vi "replace subvi from template.vi"() -> ()   [LabVIEW 2020]
uses:
  <vilib>/Utility/traverseref.llb/TRef TravTarget.ctl
  <vilib>/Utility/config.llb/Read Key (String).vi
  <vilib>/Utility/config.llb/NI_LVConfig.lvlib
  <vilib>/Utility/traverseref.llb/VI Scripting - Traverse.lvlib
panel:
  out "section exists?":bool
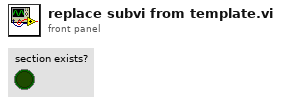
[diagram p1: front panel]
types:
  T1 = typedef "NI_LVConfig.lvlib/Config Data RefNum.ctl" = refnum<k1>
  T2 = typedef "TRef TravTarget.ctl" = enum16{"FP", "BD", "Other"}
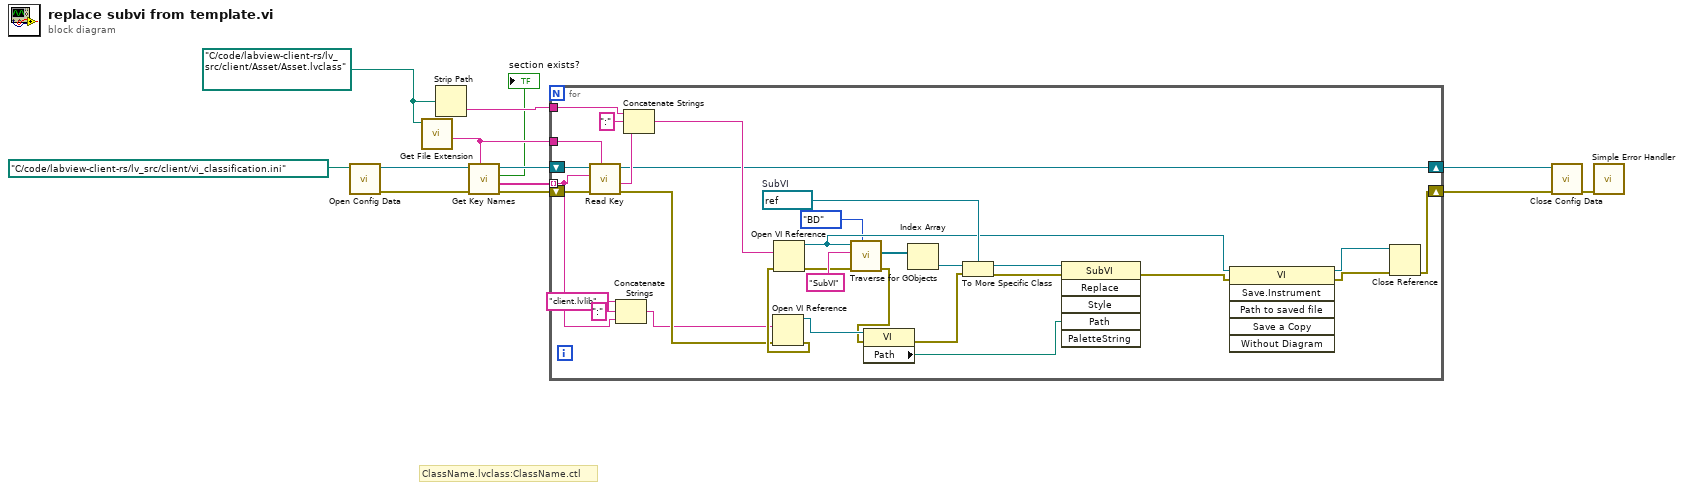
[diagram p0: block diagram]
diagram:
  w8 = path "C:/code/labview-client-rs/lv_src/client/Asset/Asset.lvclass" ("Path")
  # "ClassName.lvclass:ClassName.ctl"
  n1 = call <vilib>:"Open Config Data.vi"("configuration file path"=path "C:/code/labview-client-rs/lv_src/client/vi_classification.ini") -> ("error out"=w11:errorcluster, "refnum"=w1:T1)  [unwired: 8 in, 1 out]
  n2 = call <vilib>:"Get File Extension.vi"("file"=w8) -> ("filename without extension"=w7:string)  [unwired: 6 in, 4 out]
  n3 = Strip Path(path=w8) -> (name=w5:string)  [unwired: 1 out]
  n4 = call <vilib>:"Get Key Names.vi"("section"=w7, "error in (no error)"=w11, "refnum"=w1) -> ("error out"=w6:errorcluster, "key names"=w10:string[], "section exists?"=→"section exists?":bool, "refnum out"=w9:T1)  [unwired: 5 in]
  n5 = for {
    tunnel: w10 -> [w17] mode=indexing
    tunnel: w7 -> [w43]
    tunnel: w5 -> [w41]
    shift-right: [w25] -> w4
    shift-left: w9 -> [w44]
    shift-right: [w24] -> w3
    shift-left: w6 -> [w42]
    w34 = refnum<vi> refnum  # SubVI
    n6 = call-poly <vilib>:"Read Key.vi"("section"=w43, "error in (no error)"=w42, "key"=w17, "refnum"=w44) -> ("error out"=w18:errorcluster, "value"=w39:string, "refnum out"=w25:T1)  [unwired: 4 in, 1 out]
    n7 = Concatenate Strings("client.lvlib" ("string"), ":" ("string"), w17) -> (w14:string)
    n8 = Concatenate Strings(w41, ":" ("string"), w39) -> (w38:string)
    n9 = Open VI Reference(vi path=w14, error in (no error)=w18) -> (vi reference=w32:refnum<vi>, error out=w19:errorcluster)  [unwired: 4 in]
    n10 = Open VI Reference(vi path=w38, error in (no error)=w19) -> (vi reference=w29:refnum<vi>, error out=w20:errorcluster)  [unwired: 4 in]
    n11 = call <vilib>:"Traverse for GObjects.vi"("Traverse Target"=TRef_TravTarget."BD", "error in (no error)"=w20, "Class Name"="SubVI", "VI Refnum"=w29) -> ("error out"=w21:errorcluster, "References"=w36:refnum<vi>[])  [unwired: 4 in, 2 out]
    n12 = property class="VI"(reference=w32, error in=w21) -> (error out=w22:errorcluster, "Path"=w31:path)  [unwired: 1 out]
    n13 = Index Array(array=w36) -> (element=w35:refnum<vi>)  [unwired: 1 in]
    n14 = To More Specific Class(target class=w34, reference=w35, error in=w22) -> (specific class reference=w33:refnum<vi>, error out=w23:errorcluster)
    n15 = invoke class="SubVI" method="Replace"(reference=w33, error in=w23, "Path"=w31) -> (error out=w30:errorcluster)  [unwired: 3 in, 5 out]
    n16 = invoke class="VI" method="Save.Instrument"(reference=w29, error in=w30) -> (reference out=w27:refnum<vi>, error out=w28:errorcluster)  [unwired: 4 in, 4 out]
    n17 = Close Reference(reference=w27, error in (no error)=w28) -> (error out=w24:errorcluster)
  }
  n18 = call <vilib>:"Close Config Data.vi"("error in (no error)"=w3, "refnum"=w4) -> ("error out"=w13:errorcluster)  [unwired: 8 in, 1 out]
  n19 = call <vilib>:"Simple Error Handler.vi"("error in (no error)"=w13) -> ()  [unwired: 4 in, 5 out]
